vi "Read.vi"(8 "Error In":errorcluster, 9 "DO Channel":u8, 10 "DI Channel":u8, 11 "LINX Resource":T1) -> (0 "Error Out":errorcluster, 1 "Centimeters":dbl, 2 "Inches":dbl, 3 "LINX Resource":T1)   [LabVIEW 2020, in "LMH-LINX.lvlib" / "Ultrasonic.lvlib"]
uses:
  Ultrasonic.lvlib
  Private/Type Defs/LINX Ref.ctl
  Private/Type Defs/Platform.ctl
  Private/Type Defs/Interface.ctl
  Private/Device/Type Defs/LINX Device Config.ctl
  Private/Device/Type Defs/TCP Config.ctl
  Private/Device/Type Defs/Channels.ctl
  LMH-LINX.lvlib
  Private/Device/Device.lvlib
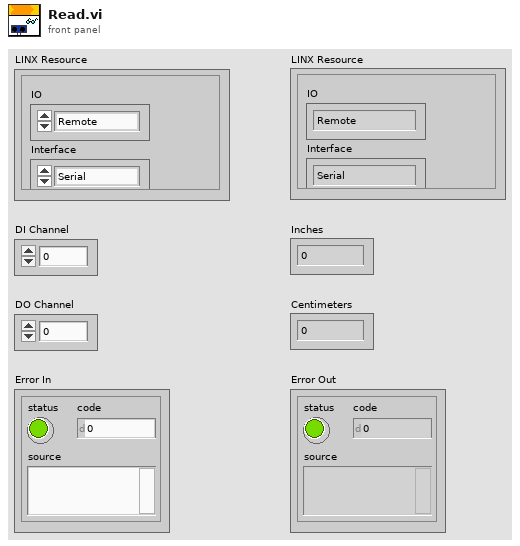
[diagram p1: front panel]
types:
  T1 = typedef "LMH-LINX.lvlib/LINX Ref.ctl" = cluster{"IO":T2, "Interface":T3, "LINX Device Config":T4}
  T2 = typedef "LMH-LINX.lvlib/Platform.ctl" = enum16{"Remote", "Local"}
  T3 = typedef "LMH-LINX.lvlib/Interface.ctl" = enum16{"Serial", "TCP"}
  T4 = typedef "Device.lvlib/LINX Device Config.ctl" = cluster{"Interface":T3, "COM Port":refnum<visa-resource-name>, "TCP Configuration":T5, "Device Family":u8, "Device ID":u8, "Device Name":string, "TCP Ref":refnum<k5>, "Channels":T6}
  T5 = typedef "Device.lvlib/TCP Config.ctl" = cluster{"IP Address":string, "Port":u16}
  T6 = typedef "LMH-LINX.lvlib/Channels.ctl" = cluster{"DI":u8[], "DO":u8[], "AI":u8[], "AO":u8[], "PWM":u8[], "QE":u8[], "UART":u8[], "I2C 2":u8[], "SPI":u8[], "CAN":u8[], "Servo":u8[], "AI Ref (V)":dbl, "AI Resolution (Bits)":u8, "AO Ref (V)":dbl, "AO Resolution (Bits)":u8}
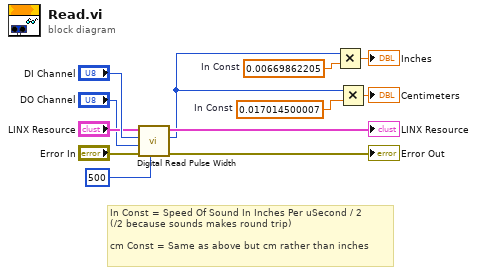
[diagram p0: block diagram]
diagram:
  w2 = 0.017014500007  # In Const
  w6 = 0.00669862205  # In Const
  # "In Const = Speed Of Sound In Inches Per uSecond / 2\n(/2 because sounds makes round trip)\n\ncm Const = Same as above but cm rather than inches"
  n1 = call "Digital Read Pulse Width.vi"("Timeout  (250 mS)"=u32 500, "Error In"="Error In", "DO Channel"="DO Channel", "DI Channel"="DI Channel", "LINX Resource"="LINX Resource") -> ("Error Out"=→"Error Out":errorcluster, "Pulse Width (uS)"=w3:u32, "LINX Resource"=→"LINX Resource":T1)  [unwired: 4 in]
  n2 = Multiply(x=w3, y=w6) -> (x*y=→"Inches":dbl)
  n3 = Multiply(x=w3, y=w2) -> (x*y=→"Centimeters":dbl)
